vi "destroyStopEvent.vi"(8 "error in (no error)":errorcluster {"code" format="Error %.0f"}, 11 "stopEventRef":T1) -> (0 "error out":errorcluster {"code" format="Error %.0f"})   [LabVIEW 2017, in "User Event - Stop.lvlib"]
doc: "Destroy the user event, even if there is an incoming error."
uses:
  User Event - Stop.lvlib
  stopEvent.ctl
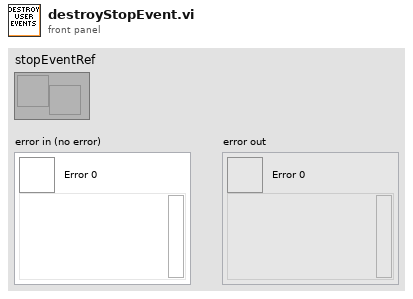
[diagram p1: front panel]
types:
  T1 = typedef "User Event - Stop.lvlib/stopEvent.ctl" = refnum<user-event>
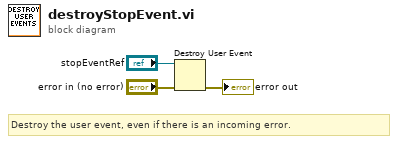
[diagram p0: block diagram]
diagram:
  # "Destroy the user event, even if there is an incoming error."
  n1 = Destroy User Event(user event="stopEventRef", error in="error in (no error)") -> (error out=→"error out":errorcluster)
